vi "AlliGator Get Phasor Harmonics, Names & Current Description.vi"(8 "Error In":errorcluster) -> (0 "Error Out":errorcluster, 1 "Current Phasor Harmonic Parameter Strings":string[](array[string]), 2 "Current Phasor Harmonics":i32[](array[numeric]), 3 "Phasor Harmonics Names":string[](array[string]), 4 "Phasor Harmonic Fequency Informations":T1[](array[typedef]) {"Base Frequency" format="%#_5g"; "Phasor Frequency" format="%#_5g"}, 5 "Dataset File Paths":path[](array[path]))   [LabVIEW 2021]
uses:
  Phasor/Phasor Harmonic Frequency Information.ctl
  Phasor/Phasor Harmonic Data.ctl
  AlliGator Variables List.ctl
  Variant/Variant to Data/Variant to [I32].vi
  AlliGator Globals, Variables & Constants.lvlib
  Variant/Variant to Data/Variant to Data.lvlib
  Phasor/Phasor.lvlib
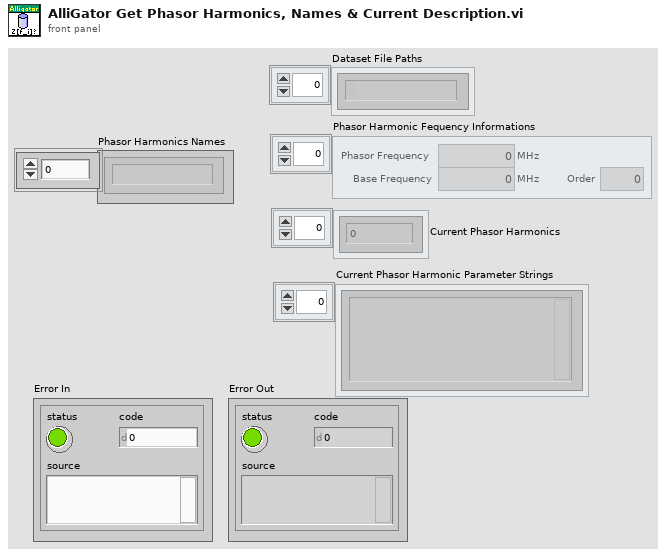
[diagram p1: front panel]
types:
  T1 = typedef "Phasor.lvlib/Phasor Harmonic Frequency Information.ctl" = cluster{"Phasor Frequency":dbl[unit], "Base Frequency":dbl[unit], "Order":u8}
  T2 = typedef "AlliGator Globals, Variables & Constants.lvlib/AlliGator Variables List.ctl" = enum16{"---- GUI ----", "Initialization Status", "State Indicators Refnum", "Original AlliGator Menu Items", "Current Action Loop State", "Script in progress", "Playback", "Loop Playback", "Search ROI Used", "Search ROI", "Decay Graph Max Legend Size", "Intensity Graph Max Legend Size", "Decay Statistics Graph Max Legend Size", "Phasor Graph Max Legend Size", "Phasor Ratio Graph Max Legend Size", "Lifetime Graph Max Legend Size", "---- Files ----", "Export Dataset Frames as Individual Files", "Show Batch Export Help Balloons", "Frames in Dataset", "ptu File Frame Start Indices", "Current Frame in Dataset", "Current Frame Timestamp", "------ Python Plugins ------", "Python Plugins Information", "Python Session", "Valid Python Session?", "---- Source Image ----", "Dataset Loaded", "Dataset Metadata", "Dataset Channel", "Dataset Data Description", "Background Dataset Metadata", "Background Dataset Channel", "Background Dataset Data Description", "Background File Subtraction", "Background File Path", "Background File Pile-up Correction", "Background File Pixel Well Capacity", "Background File Scaling Factor", "Source Image ROIs", "Current Source Image ROI", "Source Image ROI Event Refnum", "X_Source Image Display Range", "X_Source Image Palette Information", "Source Image Palette List", "Source Image Scale", "Current Dataset Load Settings", "Source Image:ROI Overlay Color", "---- Image Profile Window ----", "Image Profile:Overlay ROI in Source Image", "Image Profile Window Event Refnum", "Image Profile:IntensityType", "Image Profile:Intensity Average Type", "Image Profile:Intensity-weighted SDV", "Image Profile:Box Profile Type", "Image Profile Window Open", "Image Profile:Plotted Fit Parameter", "X_Type of Displayed Image", "X_Time Gate Slider", "Dataset Path", "Source Image Overlay to Erase", "Is Displayed Image Accumulated", "White Light Image Modified", "Mask Image Modified", "Macrotime Gate Separation", "------ Phasor Graph -------", "Phasor Graph:Show Line", "---- Phasor Plot ---", "Phasor Plot Parameters Changed", "FLI Dataset Modified since last Phasor Plot Calculation", "Phasor Harmonics Data", "Selected Phasor Harmonics", "Phasor Harmonic Manager Event Refnum", "Phasor Plot ROIs", "Current Phasor Plot ROI", "Phasor Plot ROI Event Refnum", "Phasor Plot Image Reference Points", "Phasor Plot Computed", "Phasor Plot Palette Information", "Phasor Plot Palette List", "Phasor Ratio Palette Information", "Phasor Ratio Palette List", "Phasor Image Scale", "Phasor Plot Image Overlay to Erase", "Phasor Plot Image Elements to Update", "Current Phasor Plot Calculation Parameters", "Current Phasor Calibration Options", "Reset Cumulated Phasor Plot", "Phasor Ratio Reference 1", "Phasor Ratio Lifetime Reference 1", "Phasor Ratio Reference 1 Frequency", "Phasor Ratio Reference 2", "Phasor Ratio Lifetime Reference 2", "Phasor Ratio Reference 2 Frequency", "---- Decay Analysis ----", "Number of Selected Decays to Fit", "LS Fit Results", "LAR Fit Results", "BS Fit Results", "Last Decay Max - Min", "Best Fit Parameters", "Best Fit Parameter Names", "Actual Size X", "Actual Size Y", "Binning X", "Binning Y", "Actual # Gates", "Dataset Number", "Gates to...", "Gates Skipped", "Gates to keep", "Gate Step", "Gate Separation", "Reversed Gates", "Pile-up Correction", "Pixel Well Capacity", "Background Subtracted", "Background Subtraction Method", "Background Definition Range", "Background File (deprecated)", "Number of Dataset Accumulated", "Array of Accumulated Dataset Paths", "Do Averaged Datasets", "Destination File Path", "Process Plot Target", "Use 1/D as Phasor Frequency", "---- Decay Fit Parameter Map -----", "Decay Fit Parameter Map Palette Information", "Decay Fit Parameter Map Palette List", "Local Decay Graph Window Event Refnum", "------- Local Decay Window ---------", "Use normalized IRF for convolution", "----- Miscellaneous ----", "Skippable Dialog Windows Status"}
  T3 = typedef "Phasor.lvlib/Phasor Harmonic Data.ctl" = cluster{"Phasor Harmonic Name":string, "Phasor Plot Settings Checksum":u64, "Phasor Frequency":dbl[unit], "Base Frequency":dbl[unit], "Harmonic Order":u8, "Phasor Plot Parameters":string, "Phasor Array [[CSG]]":csg[][], "Dataset File Path":path}
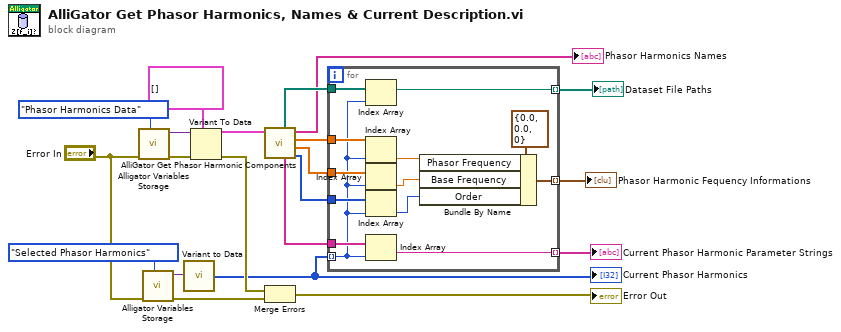
[diagram p0: block diagram]
diagram:
  n1 = call "Alligator Variables Storage.vi"("AlliGator Variable"=AlliGator_Variables_List."Phasor Harmonics Data" ("Alligator Variable"), "Error In"="Error In") -> ("Error Out"=w18:errorcluster, "Data out"=w17:variant)  [unwired: 7 in, 1 out]
  n2 = call "Alligator Variables Storage.vi"("AlliGator Variable"=AlliGator_Variables_List."Selected Phasor Harmonics" ("Alligator Variable"), "Error In"="Error In") -> ("Error Out"=w13:errorcluster, "Data out"=w21:variant)  [unwired: 7 in, 1 out]
  n3 = call-poly "Variant to Data.vi"("Variant"=w21) -> ("Value"=w4:i32[])  [unwired: 8 in]
  "Current Phasor Harmonics" <- w4
  n4 = Variant To Data(error in=w18, type=T3[] [] ("Stored ROIs in"), Variant=w17) -> (data=w11:T3[], error out=w14:errorcluster)
  n5 = call "AlliGator Get Phasor Harmonic Components.vi"("Stored Phasor Harmonics"=w11) -> ("Phasor Harmonic Orders"=w6:u8[], "Phasor Harmonic Base Fequencies"=w7:dbl[unit][], "Phasor Harmonic Frequencies"=w8:dbl[unit][], "Phasor Harmonic Names"=→"Phasor Harmonics Names":string[], "Phasor Harmonic Parameter Strings"=w10:string[], "Phasor Harmonic Dataset File Paths"=w5:path[])  [unwired: 4 in, 1 out]
  n6 = Merge Errors(w14, w13) -> (→"Error Out":errorcluster)
  n7 = for {
    tunnel: w10 -> [w34]
    tunnel: [w33] -> w9 mode=indexing
    tunnel: w8 -> [w32]
    tunnel: w7 -> [w31]
    tunnel: w6 -> [w30]
    tunnel: w5 -> [w29]
    tunnel: w4 -> [w22] mode=indexing
    tunnel: [w28] -> w3 mode=indexing
    tunnel: [w24] -> w2 mode=indexing
    n8 = Index Array(array=w29, index=w22) -> (element=w28:path)
    n9 = Index Array(array=w32, index=w22) -> (element=w27:dbl[unit])
    n10 = Index Array(array=w31, index=w22) -> (element=w26:dbl[unit])
    n11 = Index Array(array=w30, index=w22) -> (element=w25:u8)
    n12 = Index Array(array=w34, index=w22) -> (element=w33:string)
    n13 = Bundle By Name(cluster=T1 {"Phasor Frequency"=0.0, "Base Frequency"=0.0, "Order"=0} ("Phasor Harmonic Fequency Information"), "Phasor Frequency"=w27, "Base Frequency"=w26, "Order"=w25) -> (w24:T1)
  }
  "Current Phasor Harmonic Parameter Strings" <- w9
  "Phasor Harmonic Fequency Informations" <- w2
  "Dataset File Paths" <- w3
